vi "SymbolSYN.vi"() -> ()   [LabVIEW 2013]
panel:
  in  "Symbol SYN":bool
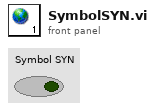
[diagram p1: front panel]
diagram:
